vi "SubVI_Acc_Filter2.vi"(8 "error in (no error)":errorcluster caption="err in", 11 "Q_data":T1) -> (0 "err out":errorcluster)   [LabVIEW 2016]
uses:
  Ctrls/raw Q data.ctl
  <vilib>/Analysis/2dsp.llb/Integral Method.ctl
  <vilib>/Analysis/8numeric.llb/1D Numeric Integration.vi
  <vilib>/measure/mascope.llb/Amplitude and Levels 1 chan.vi
  <vilib>/measure/mascope.llb/Transition Measurements 1 chan.vi
  <vilib>/measure/mamon.llb/Trigger Detection for 1 Channel.vi
  <vilib>/Waveform/WDTOps.llb/WDT Get Waveform Subset DBL.vi
  <vilib>/measure/NI_MAPro.lvlib
  <vilib>/Analysis/NI_AALPro.lvlib
panel:
  in  "Shock duration pecent [%]":u16
  in  "Filter cutoff freq":u32
  in  "파일 경로":path
  in  "인덱스":i32
  out "최대값":dbl
  out "trigger location":dbl caption="트리거 위치" format="%.1f"
  out "acc wf":waveform(dbl)(graph)
  out "Acc_time":dbl caption="Acc time" format="%#.1p"
  out "Acc_p2p":dbl=1.6258445790000002 caption="Acc peak"
  out "Raw_acc":waveform(dbl)(graph)={"t0"=timestamp(0 s since 1904-01-01), "dt"=1e-05, "Y"=array[2000 elements]}
  out "Filtered_acc":waveform(dbl)(graph)
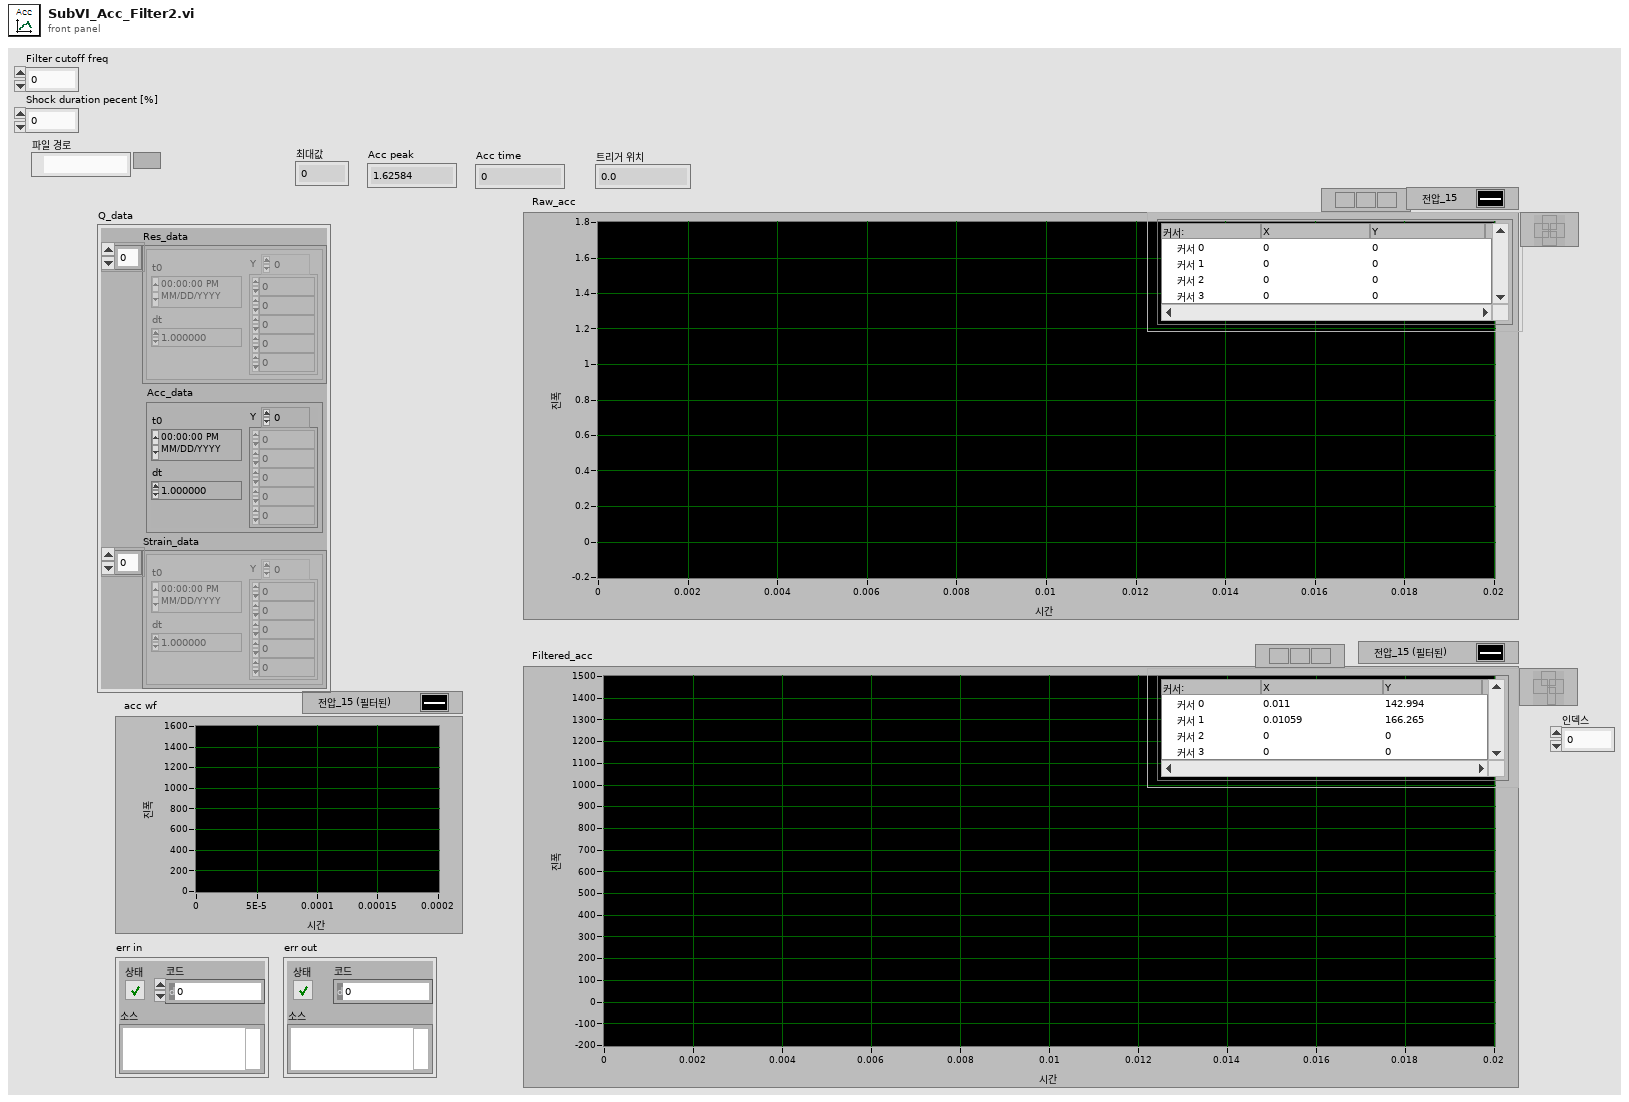
[diagram p1: front panel]
types:
  T1 = typedef "raw Q data.ctl" = cluster{"Res_data":waveform(dbl)[], "Acc_data":waveform(dbl), "Strain_data":waveform(dbl)[]}
  T2 = typedef "NI_AALPro.lvlib/Integral Method.ctl" = i32
  T3 = cluster{"method":enum32{"histogram", "peak", "auto select"}, "histogram size":i32, "histogram method":enum16{"mode"}, "reserved":dbl}
  T4 = cluster{"high ref level":dbl, "mid ref level":dbl, "low ref level":dbl, "ref units":u16}
  T5 = cluster{"Test Information":cluster{"date":string, "custom":string, "oper":string, "package":string, "pkg side":string, "solder":string, "brd side":string, "paste":string, "reflow":string}, "Sensor Set":cluster{"Accelerometer":cluster{"Sensitivity(mV/g)":dbl}, "Strain Guage":cluster{"Ch.":dbl[], "Gage factor":dbl[], "Resistance":dbl[], "Poisson ratio":dbl[]}}, "Resistor Set":cluster{"Criterion Level":dbl, "Res. Set":cluster{"Res. Ch":dbl, "Res. Active":bool, "Res Initial":dbl}[]}, "Test Stop Condition":cluster{"Test cycle":u16, "Fail number in a cycle":u16, "Fail factor":cluster{"Duration":u16, "Fail No.":u16}}, "Acceleration Condition ":cluster{"Shock duration pecent [%]":u16, "Filter cutoff freq":u32}, "Save":cluster{"Save Path":path, "File Name":string}}
  T6 = cluster{"start time":dbl, "end time":dbl, "ref levels":cluster{"high ref level":dbl, "mid ref level":dbl, "low ref level":dbl, "ref units":u16}}
  T7 = typedef "ui ctrl ref2.ctl" = cluster{"Trigger cm":refnum<vi>, "Speed In/s":refnum<vi>, "Start / Stop":refnum<vi>, "Test Information":refnum<vi>, "STATUS":refnum<vi>, "Result Table":refnum<vi>, "Acc. & Strian Result":refnum<vi>, "Curr Resistor (Ω)":refnum<vi>, "Scroll":refnum<vi>, "All Data Graph":refnum<vi>, "Acc. Graph":refnum<vi>}
  T8 = typedef "Total data.ctl" = cluster{"Raw Data":T1, "Resister result data":T9, "Result Table update":cluster{"Num":u32[], "Resister 1~5":u8[][], "Resister 6~10":u8[][], "Resister 11~15":u8[][]}, "Strain Data":cluster{"Strain 1":dbl, "Strain 2":dbl, "Strain 3":dbl, "Strain 4":dbl}, "Acc Result":cluster{"Acc Peak":dbl, "Acc time":dbl, "Acc area":dbl}, "STATUS":cluster{"status":string, "all_fail":bool, "emg":bool, "cycle":u16, "file name":string}, "Speed":dbl, "Acc peak time":dbl, "Max Strain":dbl, "Resistor at peak":cluster{"[0]":dbl, "[1]":dbl, "[2]":dbl, "[3]":dbl, "[4]":dbl, "[5]":dbl, "[6]":dbl, "[7]":dbl, "[8]":dbl, "[9]":dbl, "[10]":dbl, "[11]":dbl, "[12]":dbl, "[13]":dbl, "[14]":dbl}, "Acc peak index":u32, "time":string, "Cycle finish":bool, "Resistor at ini":cluster{"[0]":dbl, "[1]":dbl, "[2]":dbl, "[3]":dbl, "[4]":dbl, "[5]":dbl, "[6]":dbl, "[7]":dbl, "[8]":dbl, "[9]":dbl, "[10]":dbl, "[11]":dbl, "[12]":dbl, "[13]":dbl, "[14]":dbl}}
  T9 = typedef "raw data type.ctl" = cluster{"Resistor values":cluster{"[0]":dbl, "[1]":dbl, "[2]":dbl, "[3]":dbl, "[4]":dbl, "[5]":dbl, "[6]":dbl, "[7]":dbl, "[8]":dbl, "[9]":dbl, "[10]":dbl, "[11]":dbl, "[12]":dbl, "[13]":dbl, "[14]":dbl}, "Resistor tables":u8[], "Pass Fails":bool[]}
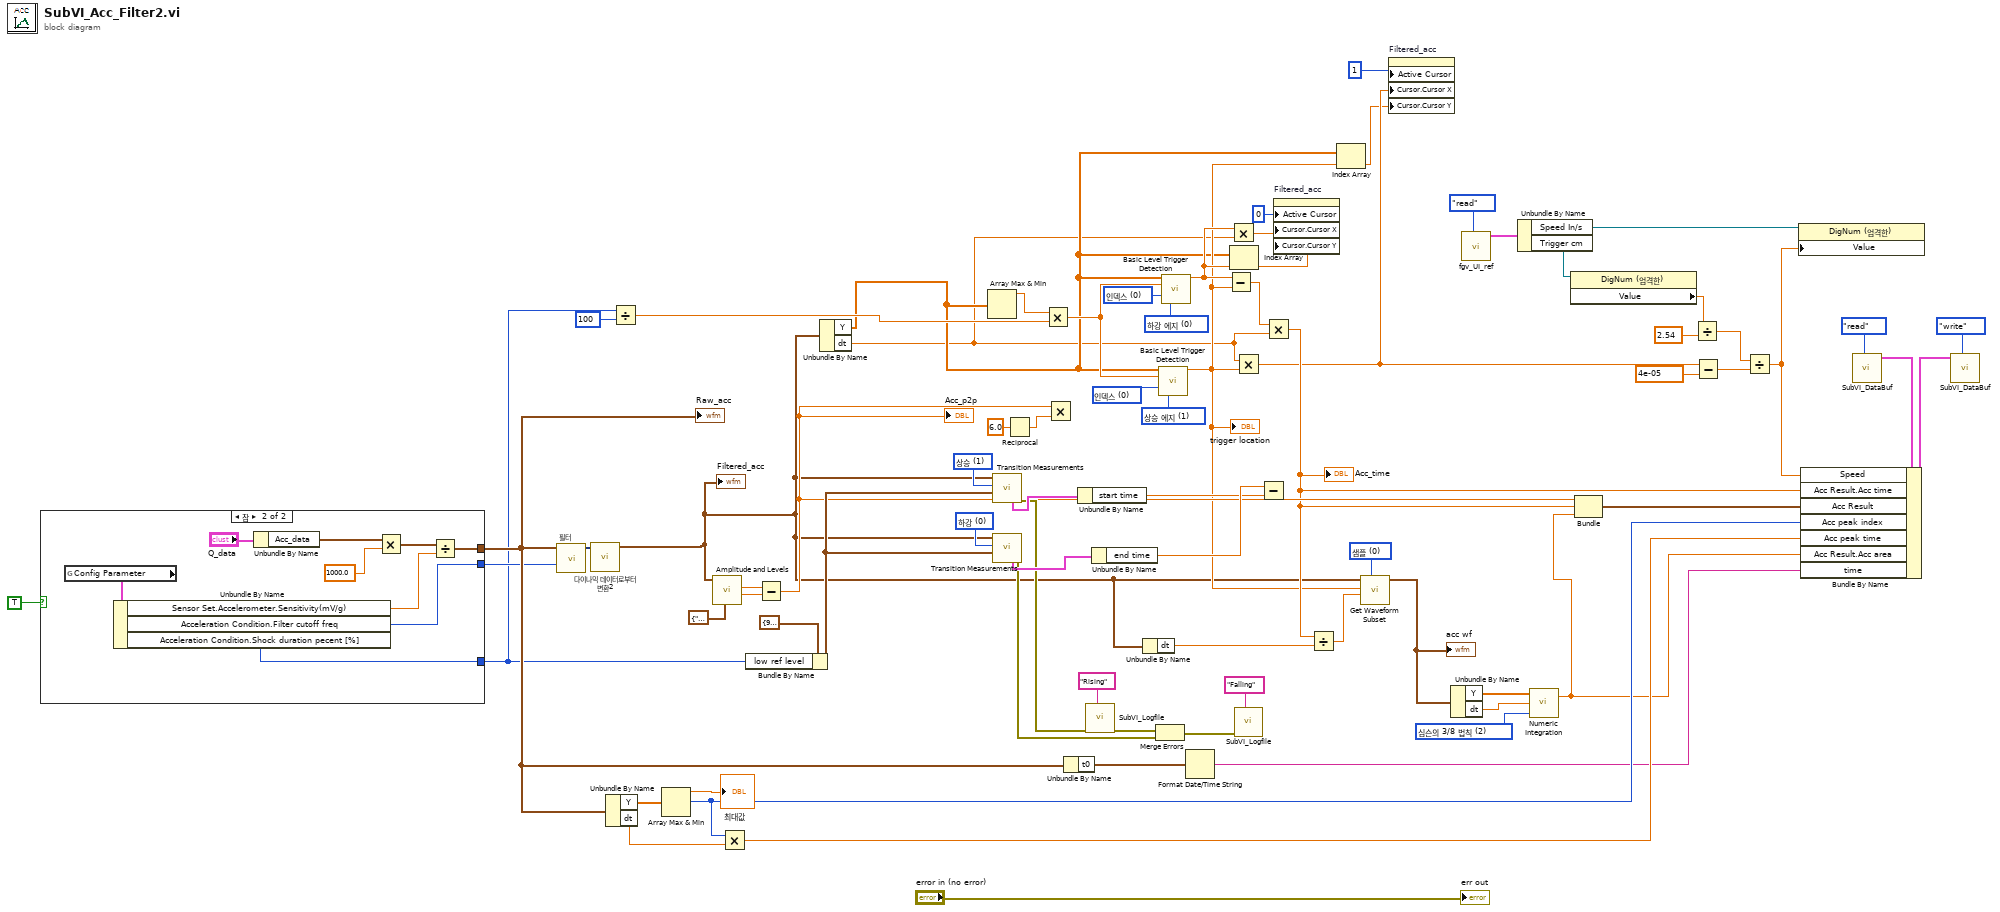
[diagram p0: block diagram]
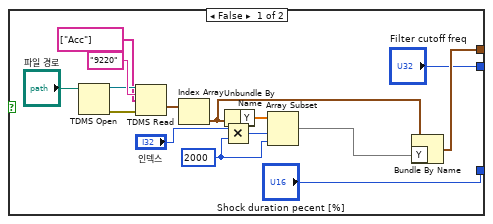
[diagram p2: hidden frame]
diagram:
  w19 = u16 0 items=["인덱스", "시간"] ("location mode")
  w20 = u16 0 items=["하강 에지", "상승 에지"] ("trigger slope")
  w43 = T2 2 items=["사다리꼴 법칙", "심슨의 법칙", "심슨의 3/8 법칙", "보데 법칙"] ("integration method")
  w52 = u16 0 items=["인덱스", "시간"] ("location mode")
  w53 = u16 1 items=["하강 에지", "상승 에지"] ("trigger slope")
  w72 = u16 0 items=["샘플 ", "상대 시간"] ("start/duration format")
  w76 = u16 0 items=["하강", "상승"] ("polarity (rising)")
  w77 = u16 1 items=["하강", "상승"] ("polarity (rising)")
  n1 = case shown="참" TRUE {
    tunnel: ["Shock duration pecent [%]" w100] -> w5
    tunnel: ["Filter cutoff freq" w93] -> w25
    tunnel: [w81 w94] -> w26
    frame False {
      w89 = 2000 ("인덱스")
      n2 = TDMS Open(11:"파일 경로") -> (0:w83:errorcluster, 3:w82:refnum<k34>)  [unwired: 6 in]
      n3 = TDMS Read(0:w82, 5:"9220" ("그룹 이름 입력"), 7:string[] ["Acc"] ("채널 이름 입력"), 11:w83) -> (10:w85:waveform(dbl)[])  [unwired: 4 in, 5 out]
      n4 = Index Array(array=w85) -> (element=w91:waveform(dbl))  [unwired: 1 in]
      n5 = Multiply(x="인덱스", y=w89) -> (x*y=w88:i32)
      n6 = Unbundle By Name(w91) -> ("Y"=w86:dbl[])
      n7 = Array Subset(array=w86, index=w88, length=w89) -> (w90:dbl[])
      n8 = Bundle By Name(cluster=w91, "Y"=w90) -> (w81:waveform(dbl))
    }
    frame True {
      n9 = global read "글로벌_Config Parameter.vi" "Config Parameter"() -> (w101:T5)
      n10 = Unbundle By Name(w101) -> ("Sensor Set.Accelerometer.Sensitivity(mV/g)"=w96:dbl, "Acceleration Condition.Filter cutoff freq"=w93:u32, "Acceleration Condition.Shock duration pecent [%]"=w100:u16)
      n11 = Unbundle By Name("Q_data") -> ("Acc_data"=w95:waveform(dbl))
      n12 = Multiply(x=w95, y=1000.0) -> (x*y=w97:waveform(dbl))
      n13 = Divide(x=w97, y=w96) -> (x/y=w94:waveform(dbl))
    }
  }
  "Raw_acc" <- w26
  n14 = call "필터"("Lower Cut-Off"=w25, "Signal"=w26) -> ("Filtered Signal"=w24:dynamicdata)  [unwired: 8 in, 1 out]
  n15 = call "다이나믹 데이터로부터 변환2"("Dynamic Data Type"=w24) -> ("Waveform"=w6:waveform(dbl))  [unwired: 3 in]
  "Filtered_acc" <- w6
  n16 = Unbundle By Name(w26) -> ("Y"=w57:dbl[], "dt"=w56:dbl)
  n17 = Divide(x=w5, y=u16 100) -> (x/y=w3:dbl)
  n18 = Array Max & Min(array=w57) -> (max value=→"최대값":dbl, max index (indices)=w54:i32)  [unwired: 2 out]
  n19 = call-poly <vilib>:"Amplitude and Levels.vi"("state settings"=T3 {"method"=enum."histogram", "histogram size"=256, "histogram method"=enum."mode", "reserved"=1.0}, "signal in"=w6) -> ("low state level"=w45:dbl, "high state level"=w44:dbl)  [unwired: 6 in, 2 out]
  n20 = Multiply(x=w54, y=w56) -> (x*y=w55:dbl)
  n21 = Bundle By Name(cluster=T4 {"high ref level"=90.0, "mid ref level"=50.0, "low ref level"=10.0, "ref units"=1} ("reference levels"), "low ref level"=w5) -> (w47:T4)
  n22 = Subtract(x=w44, y=w45) -> (x-y=w23:dbl)
  "Acc_p2p" <- w23
  n23 = Unbundle By Name(w6) -> ("Y"=w2:dbl[], "dt"=w1:dbl)
  n24 = Array Max & Min(array=w2) -> (max value=w16:dbl)  [unwired: 3 out]
  n25 = call-poly <vilib>:"Transition Measurements.vi"("reference levels"=w47, "polarity (rising)"=w77, "signal in"=w6) -> ("error out"=w33:errorcluster, "measurement info"=w75:T6)  [unwired: 3 in, 4 out]
  n26 = call-poly <vilib>:"Transition Measurements.vi"("reference levels"=w47, "polarity (rising)"=w76, "signal in"=w6) -> ("error out"=w31:errorcluster, "measurement info"=w74:T6)  [unwired: 3 in, 4 out]
  n27 = Reciprocal(x=6.0) -> (1/x=w21:dbl)
  n28 = Multiply(x=w16, y=w3) -> (x*y=w11:dbl)
  n29 = Multiply(x=w23, y=w21) -> ()  [unwired: 1 out]
  n30 = Unbundle By Name(w26) -> ("t0"=w39:timestamp)
  n31 = Unbundle By Name(w75) -> ("start time"=w64:dbl)
  n32 = call "SubVI_Logfile.vi"("Title"="Rising", "error in"=w33) -> ("error out"=w30:errorcluster)  [unwired: 9 in]
  n33 = Unbundle By Name(w74) -> ("end time"=w73:dbl)
  n34 = Unbundle By Name(w6) -> ("dt"=w36:dbl)
  n35 = Merge Errors(w30, w31) -> (w29:errorcluster)
  n36 = call-poly <vilib>:"Basic Level Trigger Detection.vi"("signal in"=w2, "level"=w11, "location mode"=w52, "trigger slope"=w53) -> ("trigger location"=w7:dbl)  [unwired: 9 in, 2 out]
  "trigger location" <- w7
  n37 = call-poly <vilib>:"Basic Level Trigger Detection.vi"("signal in"=w2, "level"=w11, "location mode"=w19, "trigger slope"=w20) -> ("trigger location"=w10:dbl)  [unwired: 9 in, 2 out]
  n38 = Format Date/Time String(seconds (now)=w39) -> (date/time string=w38:string)  [unwired: 2 in]
  n39 = Subtract(x=w10, y=w7) -> (x-y=w18:dbl)
  n40 = Multiply(x=w10, y=w1) -> (x*y=w15:dbl)
  n41 = Index Array(array=w2, index=w10) -> (element=w9:dbl)
  n42 = Multiply(x=w1, y=w7) -> (x*y=w12:dbl)
  n43 = call "SubVI_Logfile.vi"("Title"="Falling", "error in"=w29) -> ()  [unwired: 9 in, 1 out]
  n44 = Subtract(x=w73, y=w64) -> ()  [unwired: 1 out]
  n45 = Multiply(x=w18, y=w1) -> (x*y=w17:dbl)
  "Acc_time" <- w17
  n46 = property on="Filtered_acc" class="WFGraph (엄격한)"("Active Cursor"=u32 0 ("활성 커서"), "Cursor.Cursor X"=w15, "Cursor.Cursor Y"=w9) -> ()  [unwired: 2 in, 2 out]
  n47 = Divide(x=w17, y=w36) -> (x/y=w35:dbl)
  n48 = Index Array(array=w2, index=w7) -> (element=w8:dbl)
  n49 = call-poly <vilib>:"Get Waveform Subset.vi"("start/duration format"=w72, "duration"=w35, "start samples/time"=w7, "waveform in"=w6) -> ("waveform out"=w40:waveform(dbl))  [unwired: 2 in, 3 out]
  "acc wf" <- w40
  n50 = property on="Filtered_acc" class="WFGraph (엄격한)"("Active Cursor"=u32 1 ("활성 커서"), "Cursor.Cursor X"=w12, "Cursor.Cursor Y"=w8) -> ()  [unwired: 2 in, 2 out]
  n51 = Unbundle By Name(w40) -> ("Y"=w41:dbl[], "dt"=w42:dbl)
  n52 = call "fgv_UI_ref.vi"("cmd"=enum16{"write", "read"}."read") -> ("ui ref out"=w62:T7)  [unwired: 10 in]
  n53 = Unbundle By Name(w62) -> ("Speed In/s"=w61:refnum<vi>, "Trigger cm"=w60:refnum<vi>)
  n54 = call-poly <vilib>:"Numeric Integration.vi"("integration method"=w43, "dt"=w42, "Input Array"=w41) -> ("result"=w37:dbl)  [unwired: 1 out]
  n55 = property class="DigNum (엄격한)"(reference=w60) -> ("Value"=w58:dbl)  [unwired: 1 in, 2 out]
  n56 = Bundle(w23, w17, "result"=w37) -> (w67:cluster{dbl, dbl, "result":dbl})  [unwired: 1 in]
  n57 = Divide(x=w58, y=2.54) -> (x/y=w51:dbl)
  n58 = Subtract(x=w12, y=4e-05) -> (x-y=w50:dbl)
  n59 = Divide(x=w51, y=w50) -> (x/y=w49:dbl)
  n60 = property class="DigNum (엄격한)"(reference=w61, "Value"=w49) -> ()  [unwired: 1 in, 2 out]
  n61 = call "SubVI_DataBuf.vi"("cmd"=enum16{"ini", "write", "read"}."read") -> ("Total data 2"=w70:T8)  [unwired: 9 in, 1 out]
  n62 = Bundle By Name(cluster=w70, "Speed"=w49, "Acc Result.Acc time"=w17, "Acc Result"=w67, "Acc peak index"=w54, "Acc peak time"=w55, "Acc Result.Acc area"=w37, "time"=w38) -> (w66:T8)
  n63 = call "SubVI_DataBuf.vi"("cmd"=enum16{"ini", "write", "read"}."write", "Total data"=w66) -> ()  [unwired: 8 in, 2 out]
  "err out" <- "error in (no error)"
